vi "Close.vi"(8 "error in (no error)":errorcluster, 11 "Controller in":refnum<class "Panel Helper.lvclass">) -> (0 "error out":errorcluster)   [LabVIEW 2017, in "MGI-Panel Manager.lvlib" / "Panel Helper.lvclass"]
doc: "Cleans up the panel helper.\n\n----\nPlease see the following web address for additional documentation and tutorial information:\nhttp://www.mooregoodideas.com/mgi-panel-manager/\n\nAuthor: Derek Trepanier\n\nCopyright (c) 2018, Moore Good Ideas, Inc.\n\nAll rights reserved.\n\nRedistribution and use in source and binary forms, with or without modification, are permitted provided that the following conditions are met:\n\n * Redistributions of source code must retain the above copyright notice, this list of conditions and the following disclaimer.\n * Redistributions in binary form must reproduce the above copyright notice, this list of conditions and the following disclaimer in the documentation and/or other materials provided with the distribution.\n * Neither the name of Moore Good Ideas, Inc. nor the names of its contributors may be used to endorse or promote products derived from this software without specific prior written permission.\n\nTHIS SOFTWARE IS PROVIDED BY THE COPYRIGHT HOLDERS AND CONTRIBUTORS \"AS IS\" AND ANY EXPRESS OR IMPLIED WARRANTIES, INCLUDING, BUT NOT LIMITED TO, THE IMPLIED WARRANTIES OF MERCHANTABILITY AND FITNESS FOR A PARTICULAR PURPOSE ARE DISCLAIMED. IN NO EVENT SHALL THE COPYRIGHT OWNER OR CONTRIBUTORS BE LIABLE FOR ANY DIRECT, INDIRECT, INCIDENTAL, SPECIAL, EXEMPLARY, OR CONSEQUENTIAL DAMAGES (INCLUDING, BUT NOT LIMITED TO, PROCUREMENT OF SUBSTITUTE GOODS OR SERVICES; LOSS OF USE, DATA, OR PROFITS; OR BUSINESS INTERRUPTION) HOWEVER CAUSED AND ON ANY THEORY OF LIABILITY, WHETHER IN CONTRACT, STRICT LIABILITY, OR TORT (INCLUDING NEGLIGENCE OR OTHERWISE) ARISING IN ANY WAY OUT OF THE USE OF THIS SOFTWARE, EVEN IF ADVISED OF THE POSSIBILITY OF SUCH DAMAGE."
uses:
  Panel Helper.lvclass
  Deferer/Deferer.lvclass
  Panel Registry/Panel Registry.lvclass
  MGI-Panel Manager.lvlib
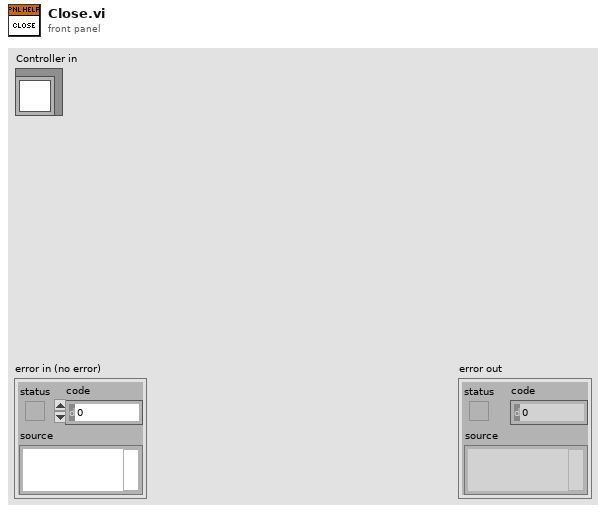
[diagram p1: front panel]
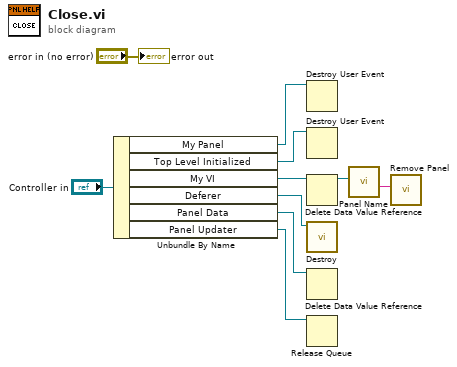
[diagram p0: block diagram]
diagram:
  n1 = Unbundle By Name("Controller in") -> ("My Panel"=w4:refnum<user-event>, "Top Level Initialized"=w9:refnum<user-event>, "My VI"=w8:refnum<data-value>, "Deferer"=w5:refnum<class "Deferer.lvclass">, "Panel Data"=w7:refnum<data-value>, "Panel Updater"=w6:refnum<queue>)
  n2 = Destroy User Event(user event=w4) -> ()  [unwired: 1 in, 1 out]
  n3 = Destroy User Event(user event=w9) -> ()  [unwired: 1 in, 1 out]
  n4 = Delete Data Value Reference(data value reference=w8) -> (data value=w2:refnum<vi>)  [unwired: 1 in, 1 out]
  n5 = call "Destroy.vi"("Deferer in"=w5) -> ()  [unwired: 10 in, 1 out]
  n6 = Delete Data Value Reference(data value reference=w7) -> ()  [unwired: 1 in, 2 out]
  n7 = Release Queue(queue=w6) -> ()  [unwired: 2 in, 3 out]
  n8 = call "Panel Name.vi"("VI in"=w2) -> ("Name"=w1:string)  [unwired: 9 in, 1 out]
  n9 = call "Remove Panel.vi"("Panel"=w1) -> ()  [unwired: 10 in, 1 out]
  "error out" <- "error in (no error)"
